vi "SaveTrack.vi"(6 "Time":dbl, 7 "Track file":path, 8 "error in (no error)":errorcluster, 9 "Focus":dbl, 10 "Y":dbl, 11 "X":dbl) -> (0 "error out":errorcluster)   [LabVIEW 2012]
uses:
  <vilib>/Utility/file.llb/Write To Spreadsheet File (DBL).vi
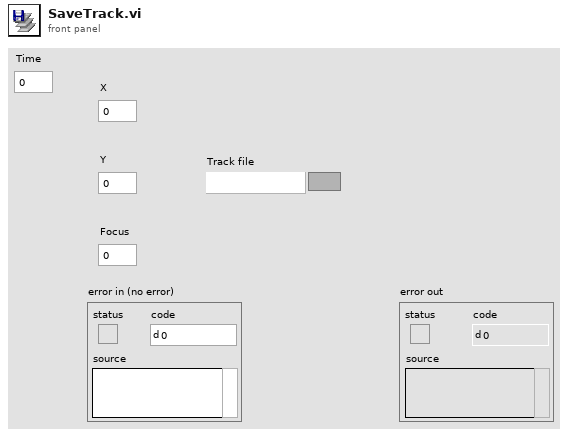
[diagram p1: front panel]
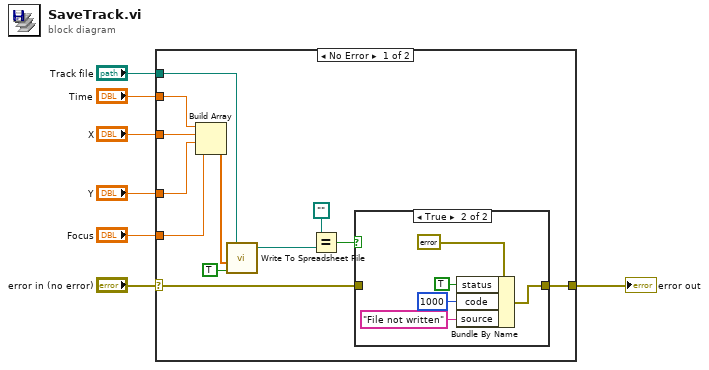
[diagram p0: block diagram]
diagram:
  n1 = case shown="No Error" "error in (no error)" {
    selector: "error in (no error)" -> [w8 w26]
    tunnel: [w9 w26] -> w6
    tunnel: "Time" -> [w19 _]
    tunnel: "X" -> [w18 _]
    tunnel: "Y" -> [w17 _]
    tunnel: "Focus" -> [w16 _]
    tunnel: "Track file" -> [w13 _]
    frame No Error {
      n2 = Build Array(w19, w18, w17, w16) -> (w15:dbl[])
      n3 = call-poly <vilib>:"Write To Spreadsheet File.vi"("append to file? (new file:F)"=TRUE, "1D data"=w15, "file path (dialog if empty)"=w13) -> ("new file path (Not A Path if cancelled)"=w11:path)  [unwired: 5 in]
      n4 = Equal?(x=path "", y=w11) -> (x = y?=w10:bool)
      n5 = case shown="True" w10 {
        tunnel: [w20 w24] -> w9
        tunnel: w8 -> [w20 _]
        frame False {
        }
        frame True {
          n6 = Bundle By Name(cluster=errorcluster {"status"=FALSE, "code"=0, "source"=""} ("error constant"), "status"=TRUE, "code"=1000, "source"="File not written") -> (w24:errorcluster)
        }
      }
    }
    frame Error {
    }
  }
  "error out" <- w6
